vi "Set Result Collector.vi"(8 "error in (no error)":errorcluster, 9 "Message Data":variant, 11 "Coverage Analyzer Process in":refnum<class "Coverage Analyzer Process.lvclass">) -> (0 "error out":errorcluster, 3 "Coverage Analyzer Process out":refnum<class "Coverage Analyzer Process.lvclass">)   [LabVIEW 2020, in "Coverage Analyzer Process.lvclass"]
uses:
  Coverage Analyzer Process.lvclass
  C:/git/astemes-lunit/source/User Interface/Process/Process.lvclass
  User Interface/Process/Process.lvclass/Process.ctl
  Coverage Analyzer Process.lvclass/Coverage Analyzer Process.ctl
  User Interface/Process/Process.lvclass
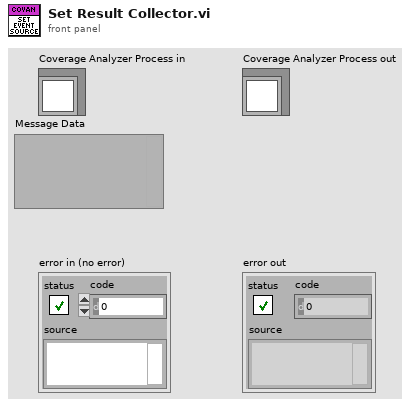
[diagram p1: front panel]
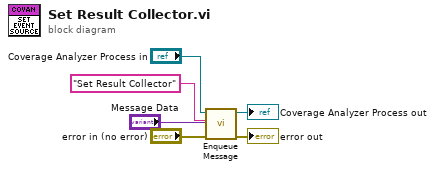
[diagram p0: block diagram]
diagram:
  n1 = call "Enqueue Message.vi"("error in (no error)"="error in (no error)", "Message Data"="Message Data", "Message"="Set Result Collector", "Process In"="Coverage Analyzer Process in") -> ("error out"=→"error out":errorcluster, "Process Out"=→"Coverage Analyzer Process out":refnum<class "Coverage Analyzer Process.lvclass">)  [unwired: 6 in]
